vi "oax_Convert Time and Speed into Transition Segments.vi"(9 "acc transition ratio":dbl, 10 "speed":dbl[](array[numeric]), 11 "time period":dbl[](array[numeric])) -> (1 "data in speed segments":T1(array[cluster]))   [LabVIEW 2017]
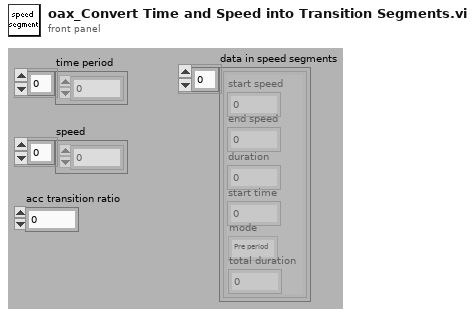
[diagram p1: front panel]
types:
  T1 = cluster{"start speed":dbl, "end speed":dbl, "duration":dbl, "start time":dbl, "mode":enum16{"Pre period", "Middle period", "Post period"}, "total duration":dbl}[]
  T2 = cluster{"Numeric":dbl, "Numeric":dbl, dbl, dbl, "enum":enum16{"Pre period", "Middle period", "Post period"}, "total duration":dbl}[]
  T3 = enum16{"Pre period", "Middle period", "Post period"}
  T4 = cluster{"Numeric":dbl, "Numeric":dbl, dbl, dbl, "enum":enum16{"Pre period", "Middle period", "Post period"}, "Numeric":dbl}
  T5 = cluster{"Numeric":dbl, "Numeric":dbl, dbl, dbl, "enum":enum16{"Pre period", "Middle period", "Post period"}, "Numeric":dbl}[]
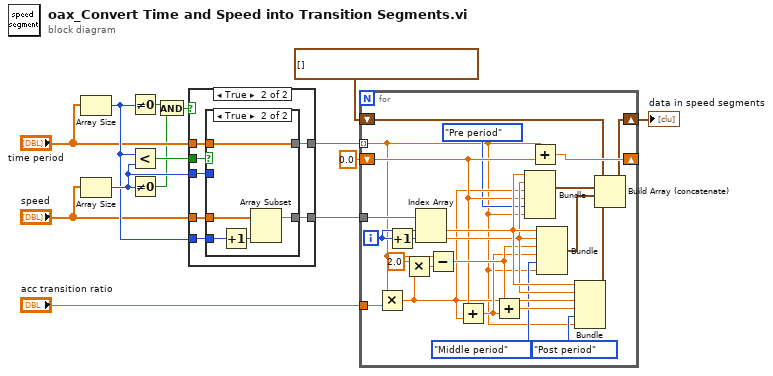
[diagram p0: block diagram]
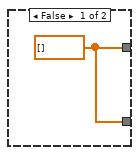
[diagram p2: hidden frame]
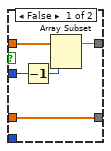
[diagram p3: hidden frame]
diagram:
  n1 = Array Size(array="time period") -> (size(s)=w8:i32)
  n2 = Array Size(array="speed") -> (size(s)=w9:i32)
  n3 = Not Equal To 0?(x=w8) -> (x != 0?=w3:bool)
  n4 = Less?(x=w8, y=w9) -> (x < y?=w6:bool)
  n5 = Not Equal To 0?(x=w9) -> (x != 0?=w4:bool)
  n6 = And(x=w3, y=w4) -> (x .and. y?=w5:bool)
  n7 = case shown="True" w5 {
    tunnel: "speed" -> [_ w22]
    tunnel: [w15 w21] -> w11
    tunnel: w6 -> [_ w20]
    tunnel: [w15 w18] -> w10
    tunnel: "time period" -> [_ w19]
    tunnel: w9 -> [_ w17]
    tunnel: w8 -> [_ w16]
    frame False {
      w15 = dbl[] []
    }
    frame True {
      n8 = case shown="True" w20 {
        tunnel: w22 -> [w24 w31]
        tunnel: [w24 w30] -> w21
        tunnel: w19 -> [w27 w32]
        tunnel: [w23 w32] -> w18
        tunnel: w17 -> [w25 _]
        tunnel: w16 -> [_ w28]
        frame False {
          n9 = Decrement(x=w25) -> (x-1=w26:i32)
          n10 = Array Subset(array=w27, length=w26) -> (w23:dbl[])  [unwired: 1 in]
        }
        frame True {
          n11 = Increment(x=w28) -> (x+1=w29:i32)
          n12 = Array Subset(array=w31, length=w29) -> (w30:dbl[])  [unwired: 1 in]
        }
      }
    }
  }
  n13 = for {
    tunnel: w10 -> [w33] mode=indexing
    tunnel: w11 -> [w55]
    shift-right: [w52] -> _
    shift-left: 0.0 -> [w43]
    tunnel: "acc transition ratio" -> [w51]
    shift-right: [w38] -> w14
    shift-left: T2 [] -> [w37]
    i -> [w54]
    n14 = Multiply(x=w33, y=w51) -> (x*y=w42:dbl)
    n15 = Increment(x=w54) -> (x+1=w53:i32)
    n16 = Multiply(x=2.0, y=w42) -> (x*y=w49:dbl)
    n17 = Index Array(array=w55, index #1=w54, index #2=w53) -> (element #1=w48:dbl, element #2=w47:dbl)
    n18 = Subtract(x=w33, y=w49) -> (x-y=w46:dbl)
    n19 = Add(x=w43, y=w42) -> (x+y=w45:dbl)
    n20 = Add(x=w46, y=w45) -> (x+y=w44:dbl)
    n21 = Bundle("Numeric"=w48, "Numeric"=w47, w42, w43, "enum"=T3."Pre period", "Numeric"=w33) -> (w41:T4)  [unwired: 1 in]
    n22 = Add(x=w33, y=w43) -> (x+y=w52:dbl)
    n23 = Bundle("Numeric"=w48, "Numeric"=w47, w46, w45, "enum"=T3."Middle period", "Numeric"=w33) -> (w40:T4)  [unwired: 1 in]
    n24 = Bundle("Numeric"=w48, "Numeric"=w47, w42, w44, "enum"=T3."Post period", "Numeric"=w33) -> (w39:T4)  [unwired: 1 in]
    n25 = Build Array (concatenate)(w37, w41, w40, w39) -> (w38:T5)
  }
  "data in speed segments" <- w14
